vi "Find Queue (SubVI).vi"(10 "Module":string, 11 "Input":T1 {"Main Config"."PR Module Configs"."Settings"."PID 2 Parameters"."output range"."output low" format="%.2f"; "Main Config"."PR Module Configs"."Settings"."PID 2 Parameters"."output range"."output high" min=0.0 max=100.0 format="%.2f"; "Main Config"."PR Module Configs"."Settings"."PID 2 Parameters"."PID gains"."derivative time (Td, min)" format="%.3f"; "Main Config"."PR Module Configs"."Settings"."PID 2 Parameters"."PID gains"."integral time (Ti, min)" format="%.3f"; "Main Config"."PR Module Configs"."Settings"."PID 2 Parameters"."PID gains"."proportional gain (Kc)" format="%.3f"; "Main Config"."Steps"."Control" items=["Pump %", "Setpoint"]; "Main Config"."TCU Module Configs"."Settings"."Huber Unistat 410 Settings"."Address" min=0 max=99 format="%02.0f"; "Main Config"."TCU Module Configs"."Settings"."Julabo FP-50 Settings"."Pump Power" min=0 max=8 step=1; "Main Config"."TCU Module Configs"."Settings"."Lauda Settings"."Pump Power" min=0 max=8 step=1; "Main Config"."Flow Module Configs"."Settings"."Bronkhorst M14 Settings"."Smoothing Steps" min=1 step=1; "Main Config"."Flow Module Configs"."Settings"."Bronkhorst M13 Settings"."Smoothing Steps" min=1 step=1; "Main Config"."Pump Module Configs"."Settings"."Ismatech 3 Channel Settings"."Channel Number" min=0 max=3; "Main Config"."Pump Module Configs"."Settings"."Ismatech 3 Channel Settings"."Pump Number" min=1; "Main Config"."Pump Module Configs"."Settings"."ASIA Pump C"."channel" min=0 max=1 step=1; "Main Config"."Pump Module Configs"."Settings"."Masterflex"."Pump Number" min=1.0 max=20.0 step=1.0; "Main Config"."Pump Module Configs"."Settings"."Ismatech"."Pump Number" min=1.0 max=20.0 step=1.0; "Main Config"."Feed Module Configs"."Settings"."Bronkhorst M14 Settings"."Smoothing Steps" min=1 step=1; "Main Config"."Feed Module Configs"."Settings"."Ismatech 3 Channel Settings"."Channel Number" min=0 max=3; "Main Config"."Feed Module Configs"."Settings"."Ismatech 3 Channel Settings"."Pump Number" min=1; "Main Config"."Feed Module Configs"."Settings"."output range"."output low" min=0.0 max=100.0 format="%.2f"; "Main Config"."Feed Module Configs"."Settings"."output range"."output high" format="%.2f"; "Main Config"."Feed Module Configs"."Settings"."PID 2 Parameters"."PID gains"."derivative time (Td, min)" format="%.3f"; "Main Config"."Feed Module Configs"."Settings"."PID 2 Parameters"."PID gains"."integral time (Ti, min)" format="%.3f"; "Main Config"."Feed Module Configs"."Settings"."PID 2 Parameters"."PID gains"."proportional gain (Kc)" format="%.3f"; "Main Config"."Feed Module Configs"."Settings"."Bronkhorst M13 Flow Meter"."Smoothing Steps" min=1 step=1; "Main Config"."Feed Module Configs"."Settings"."ASIA Pump C"."channel" min=0 max=1 step=1; "Main Config"."Feed Module Configs"."Settings"."Ismatech"."Pump Number" min=1.0 max=20.0 step=1.0; "Main Config"."Feed Module Configs"."Settings"."Masterflex"."Pump Number" min=1.0 max=20.0 step=1.0}) -> (2 "Found?":bool, 3 "Queue out":refnum<queue>)   [LabVIEW 2018, in "Sequencing Library.lvlib"]
uses:
  Sequencing Library.lvlib
  support/Message Queue/Message Cluster.ctl
  Drag and Drop/State Cluster.ctl
  Drag and Drop/Thumbnail Cluster.ctl
  Drag and Drop/Object Cluster.ctl
  <vilib>/Utility/miscctls.llb/LVRectTypeDef.ctl
  Drag and Drop/Object Type Enum.ctl
  <vilib>/Utility/miscctls.llb/LVPositionTypeDef.ctl
  Config Module/Controls/Main Config Cluster.ctl
  OPC/OPC Module Config.ctl
  Scale Module Folder/Measure Instrument/State Enum.ctl
  <vilib>/Utility/miscctls.llb/LVPoint32TypeDef.ctl
  OPC/OPC Settings.ctl
  OPC/Variable Data Cluster.ctl
  <vilib>/OPCUA/controls/NodeId.ctl
  <vilib>/OPCUA/controls/OPC UA StatusCode.ctl
  <vilib>/OPCUA/controls/Subscription ID.ctl
  <vilib>/OPCUA/controls/OPC UA Client Refnum.ctl
  <vilib>/OPCUA/controls/Subscription Data Change.ctl
  <vilib>/OPCUA/controls/Data Type.ctl
  OPC/OPC Tag Data.ctl
  Feed Module/Controls/Feed Module Config Cluster.ctl
  Feed Module/Controls/Feed Module Settings Cluster.ctl
  Ismatec ISM 831C/Controls/Ismatech ISM831C Settings Cluster.ctl
  Masterflex 7550-30/Controls/Settings Cluster.ctl
  Mettler Toledo/Controls/Settings Cluster.ctl
  Bronkhorst M13 Flow Meter/Settings Cluster.ctl
  Measure Instrument/PID 2 Parameters Cluster.ctl
  Measure Instrument/PID Input Enum.ctl
  Measure Instrument/PID 2 Output Enum.ctl
  Tacmina QI/Tacmina QI DAQ Setting.ctl
  KNF Pump/Settings Cluster plus SIMDOS.ctl
  ASIA Pump/Pump Settings.ctl
  VICI M50 Party Mode/Settings Cluster.ctl
  FLOM Pump/Settings Cluster.ctl
  SSI PR Class/SSI PR or LD Settings Cluster.ctl
  Masterflex 75211/Masterflex 75211 DAQ Setting.ctl
  SSI PR Class/SSI P40 Settings Cluster.ctl
  Ismatec 78001/Ismatec 4083.ctl
  Bronkhorst M14 Flow Meter/Settings Cluster.ctl
  TT Module/Controls/TT Module Config Cluster.ctl
  Tag VIs/Numeric Alarm Settings Cluster.ctl
  Acquisition/Hardware Configuration.ctl
  Acquisition/Task Cluster.ctl
  PT Module/Controls/PT Module Config Cluster.ctl
  Scale Module Folder/Feed Module/Controls/Scale Module Config Cluster.ctl
  Scale Module Folder/Feed Module/Controls/Scale Module Settings Cluster.ctl
  Pump Module Folder/Pump Module Config Cluster.ctl
  Pump Module Folder/Pump Module Settings Cluster.ctl
  LabJack Module/Controls/U3 Module Config Cluster.ctl
  Decoration Module/Decoration Module Config Cluster.ctl
  Flow Module Folder/Feed Module/Controls/Flow Module Config Cluster.ctl
  Flow Module Folder/Feed Module/Controls/Flow Module Settings Cluster.ctl
  TCU Module/TCU Module Folder/TCU Module Config Cluster.ctl
  TCU Module/TCU Module Folder/TCU Module Settings Cluster.ctl
  TCU Module/TCU Module Folder/Measure Instrument/Output Devices.ctl
  Huber TCU/Huber Settings.ctl
  Lauda Integral XT-150 TCU/Lauda Settings.ctl
  Julabo Type 1 TCU/Julabo Type 1 TCU Folder/Julabo FP-50 Settings.ctl
  Huber Unistat 410 TCU/Huber Unistat 410 RS485 Settings.ctl
  D-O Module Folder/Not Sure Where this is Used.ctl
  Squence Control.ctl
  D-O Module Folder/D-O Module Config Cluster.ctl
  D-O Module Folder/Valve Clusters.ctl
  D-O Module Folder/D-O Module Settings Cluster.ctl
  D-O Module Folder/D-O Device Settings Cluster.ctl
  VICI Electronic Actuator/VICI Electronic Actuator Settings.ctl
  Pressure Regulator Control Module/Pressure Regulator/Controls/4-20mA Module Config Cluster.ctl
  Pressure Regulator Control Module/Pressure Regulator/Controls/4-20mA Module Settings Cluster.ctl
  Pressure Transmitter/Pressure Transmitter Device Settings.ctl
  Pressure Reg Module/Pressure Regulator Device Settings.ctl
  Sonicator Module Folder/Feed Module/Controls/Sonicator Module Config Cluster.ctl
  Sonicator Module Folder/Feed Module/Controls/Sonicator Module Settings Cluster.ctl
  Sonic Systems P100/Sonic Systems P100 Settings.ctl
  Agitator Module Folder - Copy/Feed Module/Controls/Agitator Module Config Cluster.ctl
  Agitator Module Folder - Copy/Feed Module/Controls/Agitator Module Settings Cluster.ctl
  support/Message Queue/Message Queue.lvlib
  TT Module/TT Module.lvlib
  Ismatec ISM 831C/Ismatec ISM 831C.lvlib
  Masterflex 7550-30/Masterflex 7550-30.lvlib
  Mettler Toledo/Mettler Toledo.lvlib
  Bronkhorst M13 Flow Meter/Bronkhorst M13 Flow Meter.lvlib
  Tacmina QI/Tacmina QI.lvlib
  KNF Pump/KNF SIMDOS.lvlib
  ASIA Pump.lvlib
  Feed Module/Feed Module.lvlib
  DAQ/DAQ.lvlib
  PT Module/PT Module.lvlib
  Scale Module Folder/Scale Module.lvlib
  Pump Module Folder/Pump Module.lvlib
  LabJack Module/U3 Module.lvlib
  Flow Module Folder/Flow Module.lvlib
  Huber TCU/Huber Ministat 230 TCU.lvlib
  Lauda Integral XT-150 TCU/Lauda TCU.lvlib
  Julabo Type 1 TCU/Julabo Type 1 TCU Folder/Julabo Type FP-50 TCU.lvlib
  TCU Module/TCU Module Folder/TCU Module.lvlib
  Config Module/Config Module.lvlib
  Drag and Drop/Drag and Drop.lvlib
  VICI M50 Party Mode/VICI M6 M50 Party Mode.lvlib
  D-O Module Folder/D-O Module.lvlib
  Pressure Transmitter/Pressure Transmitter Library.lvlib
  Pressure Regulator Control Module/Pressure Regulator/4-20mA Module.lvlib
  Pressure Reg Module/Pressure Regulator Library.lvlib
  FLOM Pump/FLOM Pump.lvlib
  SSI PR Class/SSI PR or LD Pump.lvlib
  OPC/OPC UA.lvlib
  Scale Module Folder/Measure Instrument/Scale Module Engine.lvlib
  D-O Module Folder/DIO Valve/VICI Electronic Actuator.lvlib
  Masterflex 75211/Masterflex 75211.lvlib
  SSI PR Class/SSI P40 Pump.lvlib
  Huber Unistat 410 TCU/Huber Unistat 410 TCU.lvlib
  Ismatec 78001/Ismatec 4308.lvlib
  Bronkhorst M14 Flow Meter/Bronkhorst M14 Flow Meter.lvlib
  Sonicator Module Folder/Sonicator Module.lvlib
  Sonic Systems P100/Sonic Systems P100.lvlib
  Agitator Module Folder - Copy/Agitator Module.lvlib
panel:
  # "Agitator Settings"
  # "Sonicator Settings"
  # "Instrument Settings"
  # "Instrument Settings"
  # "Output Instruments"
  # "Flow Meter Settings"
  # "Output Instruments"
  # "Scale Settings"
  # "Output Instruments"
  # "Input Instruments"
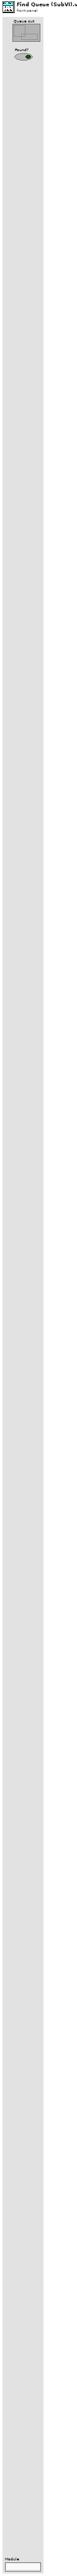
[diagram p1: front panel]
types:
  T1 = typedef "Drag and Drop.lvlib/State Cluster.ctl" = cluster{"VI refs":refnum<vi>[], "Queues":refnum<queue>[], "[Thumbnails]":T2[], "Drag Object Idx":i32, "[Objects]":T3[], "Active Object":i32, "Drop Offset":T6, "Process Name":string, "Main Config":T7, "Campaign Filepath":path, "Config Changed?":bool}
  T2 = typedef "Thumbnail Cluster.ctl" = cluster{"Path":path, "Rectangle":cluster{"left":i16, "top":i16, "right":i16, "bottom":i16}}
  T3 = typedef "Object Cluster.ctl" = cluster{"BMP Path":path, "Anchor Position":cluster{"X":i32, "Y":i32}, "Hot Spot":T4, "Type":T5, "Parameters":variant}
  T4 = typedef "LVRectTypeDef.ctl" = cluster{"Left":i16, "Top":i16, "Right":i16, "Bottom":i16}
  T5 = typedef "Object Type Enum.ctl" = enum16{"Icon", "Line", "Text", "Feed Module"}
  T6 = typedef "LVPositionTypeDef.ctl" = cluster{"Left":i32, "Top":i32}
  T7 = typedef "Config Module.lvlib/Main Config Cluster.ctl" = cluster{"Notebook":string, "OPC Module Configs":T8[], "Feed Module Configs":T18[], "Log File Path":path, "TT Module Configs":T37[], "DAQ Config":T39, "PT Module Configs":T41[], "Scale Module Configs":T42[], "Pump Module Configs":T44[], "U3 Module Configs":T46[], "Decoration Module Configs":T47[], "Flow Module Configs":T48[], "TCU Module Configs":T50[], "Steps":T57, "Abort":bool, "DO Module Configs":T59[], "PR Module Configs":T64[], "SC Module Configs":T68[], "AM Module Configs":T71[], "Cycle Period":dbl}
  T8 = typedef "OPC UA.lvlib/OPC Module Config.ctl" = cluster{"State":T9, "GUID":string, "Drop Coords":T10, "Configuration":T11, "First Iteration":bool, "Data":cluster{"Object Name":string, "Variable Array":T12[]}[], "Process Name":string, "Load Count":i32, "Log Started":bool, "subscription ID out":T15, "OPC UA client refnum out":T16, "Event Registration Refnum":refnum<event-registration>, "Start Time":timestamp, "Current Time":timestamp, "Tag Data":T17[]}
  T9 = typedef "Scale Module.lvlib/Scale Module Engine.lvlib/State Enum.ctl" = enum16{"Measuring", "Idle"}
  T10 = typedef "LVPoint32TypeDef.ctl" = cluster{"Horizontal":i32, "Vertical":i32}
  T11 = typedef "OPC UA.lvlib/OPC Settings.ctl" = cluster{"Cycle Period":dbl, "server endpoint URL":string, "security policy":cluster{"message mode":enum16{"None", "Sign", "Sign and Encrypt"}, "security":enum16{"Basic256", "Basic128Rsa15"}}, "Trust Any Server":bool}
  T12 = typedef "OPC UA.lvlib/Variable Data Cluster.ctl" = cluster{"node ID":T13, "browse name":string, "status":T14, "timestamp":timestamp, "value ":variant}
  T13 = typedef "NodeId.ctl" = string
  T14 = typedef "OPC UA StatusCode.ctl" = u32
  T15 = typedef "Subscription ID.ctl" = u32
  T16 = typedef "OPC UA Client Refnum.ctl" = refnum<k21>
  T17 = typedef "OPC UA.lvlib/OPC Tag Data.ctl" = cluster{"Include this Device":bool, "Device Name":string, "OPC Tag Data":cluster{"Tag":string, "Value":variant, "Time Stamp":timestamp}[]}
  T18 = typedef "Feed Module.lvlib/Feed Module Config Cluster.ctl" = cluster{"GUID":string, "Drop Coords":T10, "Process Name":string, "Queue Name":string, "Settings":T19, "Settings Load Count":i32, "OP Load Count":i32}
  T19 = typedef "Feed Module.lvlib/Feed Module Settings Cluster.ctl" = cluster{"Cycle Period":dbl, "Ismatech":T20, "Masterflex":T21, "Mettler":T22, "Bronkhorst M13 Flow Meter":T23, "PID 2 Parameters":T24, "Manual Entry":dbl, "Auto?":bool, "output range":cluster{"output high":dbl, "output low":dbl}, "Tacmina Settings":T27, "KNF SIMDOS Settings":T28, "ASIA Pump C":T29, "VICI Settings":T30, "FLOM Settings":T31, "SSI PR/LD Settings":T32, "Masterflex 75211 Settings":T33, "SSI P40 Settings":T34, "Ismatech 3 Channel Settings":T35, "Bronkhorst M14 Settings":T36}
  T20 = typedef "Ismatec ISM 831C.lvlib/Ismatech ISM831C Settings Cluster.ctl" = cluster{"VISA resource name":refnum<visa-resource-name>, "Simulated?":bool, "Pump Number":dbl, "Reverse?":bool}
  T21 = typedef "Masterflex 7550-30.lvlib/Settings Cluster.ctl" = cluster{"VISA resource name":refnum<visa-resource-name>, "Simulated?":bool, "Pump Number":dbl, "Reverse?":bool}
  T22 = typedef "Mettler Toledo.lvlib/Settings Cluster.ctl" = cluster{"VISA resource name":refnum<visa-resource-name>, "Simulated?":bool}
  T23 = typedef "Bronkhorst M13 Flow Meter.lvlib/Settings Cluster.ctl" = cluster{"VISA resource name":refnum<visa-resource-name>, "Simulated?":bool, "Smoothing Steps":i32}
  T24 = typedef "PID 2 Parameters Cluster.ctl" = cluster{"Input Device":T25, "Output Device":T26, "Setpoint":dbl, "PID gains":cluster{"proportional gain (Kc)":dbl, "integral time (Ti, min)":dbl, "derivative time (Td, min)":dbl}}
  T25 = typedef "PID Input Enum.ctl" = enum16{"Default", "Bronkhorst M13", "Bronkhorst M14", "Scale Rate of Change"}
  T26 = typedef "PID 2 Output Enum.ctl" = enum16{"Default", "Ismatec ISM 4308", "Ismatec ISM 831C", "Masterflex 7550-30", "VICI", "Tacmina QI", "KNF SIMDOS", "ASIA Type C", "FLOM UI-22-11", "SSI PR/LD", "SSI P40", "Masterflex 75211-70"}
  T27 = typedef "Tacmina QI.lvlib/Tacmina QI DAQ Setting.ctl" = cluster{"Analog DAQ Task":refnum<k21>, "Digital DAQ Task":refnum<k21>}
  T28 = typedef "KNF SIMDOS.lvlib/Settings Cluster plus SIMDOS.ctl" = cluster{"VISA resource name":refnum<visa-resource-name>, "Simulated?":bool}
  T29 = typedef "ASIA Pump.lvlib/Pump Settings.ctl" = cluster{"ASIA Pump #":i32, "channel":i32, "Simulated":bool}
  T30 = typedef "VICI M6 M50 Party Mode.lvlib/Settings Cluster.ctl" = cluster{"VISA resource name":refnum<visa-resource-name>, "Simulated?":bool, "Pump Letter":string, "Reverse?":bool}
  T31 = typedef "FLOM Pump.lvlib/Settings Cluster.ctl" = cluster{"VISA resource name":refnum<visa-resource-name>, "Simulated?":bool, "Pump Number":dbl}
  T32 = typedef "SSI PR or LD Pump.lvlib/SSI PR or LD Settings Cluster.ctl" = cluster{"VISA resource name":refnum<visa-resource-name>, "Simulated?":bool}
  T33 = typedef "Masterflex 75211.lvlib/Masterflex 75211 DAQ Setting.ctl" = cluster{"Analog DAQ Task":refnum<k21>, "Digital DAQ Task":refnum<k21>}
  T34 = typedef "SSI P40 Pump.lvlib/SSI P40 Settings Cluster.ctl" = cluster{"VISA resource name":refnum<visa-resource-name>, "Simulated?":bool}
  T35 = typedef "Ismatec 4308.lvlib/Ismatec 4083.ctl" = cluster{"VISA resource name":refnum<visa-resource-name>, "Pump Number":i16, "Channel Number":i16, "Simulated?":bool, "Reverse?":bool}
  T36 = typedef "Bronkhorst M14 Flow Meter.lvlib/Settings Cluster.ctl" = cluster{"VISA resource name":refnum<visa-resource-name>, "Simulated?":bool, "Smoothing Steps":i32}
  T37 = typedef "TT Module.lvlib/TT Module Config Cluster.ctl" = cluster{"GUID":string, "Drop Coords":T10, "Input Channel Tag Name ":string, "Process Name":string, "Queue Name":string, "Input Channel Numeric Alarm Settings":T38[]}
  T38 = typedef "Numeric Alarm Settings Cluster.ctl" = cluster{"enable? (F)":bool, "name":string, "alarm type":enum16{"HI_HI", "HI", "LO", "LO_LO"}, "level/change":dbl, "deadband/time":dbl, "alarm delay":dbl, "priority":u32, "ack type":enum16{"Auto", "User", "None", "Each Occurrence"}, "area":string, "description":string, "log? (T)":bool}
  T39 = typedef "DAQ.lvlib/Hardware Configuration.ctl" = cluster{"Tasks":T40[]}
  T40 = typedef "Task Cluster.ctl" = cluster{"DAQmx Task":refnum<k21>, "Read-Write Radio":enum32{"Read", "Write"}}
  T41 = typedef "PT Module.lvlib/PT Module Config Cluster.ctl" = cluster{"GUID":string, "Drop Coords":T10, "Input Channel Tag Name ":string, "Process Name":string, "Queue Name":string, "Input Channel Numeric Alarm Settings":T38[]}
  T42 = typedef "Scale Module.lvlib/Scale Module Config Cluster.ctl" = cluster{"GUID":string, "Drop Coords":T10, "Process Name":string, "Queue Name":string, "Settings":T43, "Load Count":i32}
  T43 = typedef "Scale Module.lvlib/Scale Module Settings Cluster.ctl" = cluster{"Cycle Period":dbl, "Mettler":T22, "Scale Type":string}
  T44 = typedef "Pump Module.lvlib/Pump Module Config Cluster.ctl" = cluster{"GUID":string, "Drop Coords":T10, "Process Name":string, "Queue Name":string, "Settings":T45, "Load Count":i32}
  T45 = typedef "Pump Module.lvlib/Pump Module Settings Cluster.ctl" = cluster{"Cycle Period":dbl, "Manual Entry":dbl, "Output Device":T26, "Ismatech":T20, "Ismatech 3 Channel Settings":T35, "Masterflex":T21, "VICI Settings":T30, "Tacmina Settings":T27, "KNF SIMDOS Settings":T28, "ASIA Pump C":T29, "FLOM Settings":T31, "SSI PR/LD Settings":T32, "SSI P40 Settings":T32, "Masterflex 75211 Settings":T33, "Pump Calibration File":path, "Calibration Slope":dbl, "Calibration Y Intercept":dbl, "Pump Cal Enum":u16}
  T46 = typedef "U3 Module.lvlib/U3 Module Config Cluster.ctl" = cluster{"GUID":string, "Drop Coords":T10, "AI Channel Number":enum16{"Default", "AI0", "AI1", "AI2", "AI3", "AI4", "AI5", "AI6", "AI7"}, "Process Name":string, "Queue Name":string, "Input Channel Numeric Alarm Settings":T38[]}
  T47 = typedef "Decoration Module Config Cluster.ctl" = cluster{"GUID":string, "Drop Coords":T10, "Decoration Filepath":path}
  T48 = typedef "Flow Module.lvlib/Flow Module Config Cluster.ctl" = cluster{"GUID":string, "Drop Coords":T10, "Process Name":string, "Queue Name":string, "Settings":T49, "Load Count":i32}
  T49 = typedef "Flow Module.lvlib/Flow Module Settings Cluster.ctl" = cluster{"Cycle Period":dbl, "Flow Meter Type":string, "Bronkhorst M13 Settings":T23, "Bronkhorst M14 Settings":T36}
  T50 = typedef "TCU Module.lvlib/TCU Module Config Cluster.ctl" = cluster{"GUID":string, "Drop Coords":T10, "Process Name":string, "Queue Name":string, "Settings":T51, "Load Count":i32, "Power Level Changed":bool}
  T51 = typedef "TCU Module.lvlib/TCU Module Settings Cluster.ctl" = cluster{"Cycle Period":dbl, "Setpoint Entry":dbl, "Output Device":T52, "Huber Ministat 230 Settings":T53, "Lauda Settings":T54, "Julabo FP-50 Settings":T55, "Internal Control?":bool, "Huber Unistat 410 Settings":T56}
  T52 = typedef "Output Devices.ctl" = enum16{"Default", "Huber Ministat 230", "Huber Unistat 410", "Lauda XT-150", "Julabo FP-50"}
  T53 = typedef "Huber Ministat 230 TCU.lvlib/Huber Settings.ctl" = cluster{"VISA resource name":refnum<visa-resource-name>, "Simulated?":bool}
  T54 = typedef "Lauda TCU.lvlib/Lauda Settings.ctl" = cluster{"VISA resource name":refnum<visa-resource-name>, "Simulated?":bool, "Pump Power":i32}
  T55 = typedef "Julabo Type FP-50 TCU.lvlib/Julabo FP-50 Settings.ctl" = cluster{"VISA resource name":refnum<visa-resource-name>, "Simulated?":bool, "Pump Power":i32}
  T56 = typedef "Huber Unistat 410 TCU.lvlib/Huber Unistat 410 RS485 Settings.ctl" = cluster{"VISA resource name":refnum<visa-resource-name>, "Address":i8, "Simulated?":bool}
  T57 = typedef "Not Sure Where this is Used.ctl" = T58[]
  T58 = typedef "Sequencing Library.lvlib/Squence Control.ctl" = cluster{"Module":string, "Control":u16, "Value":dbl, "Wait (sec)":dbl}
  T59 = typedef "D-O Module.lvlib/D-O Module Config Cluster.ctl" = cluster{"GUID":string, "Drop Coords":T10, "Process Name":string, "Queue Name":string, "Settings":T60, "Load Count":i32}
  T60 = typedef "D-O Module.lvlib/Valve Clusters.ctl" = cluster{"Valve Settings":T61, "Valve Type":enum16{"Default", "Digital Output Valve", "VICI Electronic Actuator"}, "Time On (Sec)":dbl, "Time Off (Sec)":dbl, "Run?":bool}
  T61 = typedef "D-O Module.lvlib/D-O Module Settings Cluster.ctl" = cluster{"D-O Settings":T62, "VICI Electronic Actuator":T63}
  T62 = typedef "D-O Module.lvlib/D-O Device Settings Cluster.ctl" = cluster{"DAQmx Task Name":refnum<k21>, "Output Channel":u16, "Output Channel Names":string[]}
  T63 = typedef "VICI Electronic Actuator.lvlib/VICI Electronic Actuator Settings.ctl" = cluster{"VISA resource name":refnum<visa-resource-name>, "Mode":enum16{"Two Positions With Stops", "Two Positions Without Stops", "Mutiposition"}, "Simulated":bool}
  T64 = typedef "4-20mA Module.lvlib/4-20mA Module Config Cluster.ctl" = cluster{"GUID":string, "Drop Coords":T10, "Process Name":string, "Queue Name":string, "Settings":T65, "Settings Load Count":i32}
  T65 = typedef "4-20mA Module.lvlib/4-20mA Module Settings Cluster.ctl" = cluster{"Cycle Period":dbl, "PID 2 Parameters":cluster{"Input Device":enum16{"Default", "4-20mA"}, "Output Device":enum16{"Default", "Equilibar Pressure Reg", "Flow Regulator"}, "Setpoint":dbl, "PID gains":cluster{"proportional gain (Kc)":dbl, "integral time (Ti, min)":dbl, "derivative time (Td, min)":dbl}, "output range":cluster{"output low":dbl, "output high":dbl}}, "Manual Entry":dbl, "Auto?":bool, "4-20mA Input Settings":T66, "4-20mA Out Settings":T67, "Input Channel Tag Name ":string}
  T66 = typedef "Pressure Transmitter Library.lvlib/Pressure Transmitter Device Settings.ctl" = cluster{"Input Channel ":u16}
  T67 = typedef "Pressure Regulator Library.lvlib/Pressure Regulator Device Settings.ctl" = cluster{"Output DAQ Task":refnum<k21>}
  T68 = typedef "Sonicator Module.lvlib/Sonicator Module Config Cluster.ctl" = cluster{"GUID":string, "Drop Coords":T10, "Process Name":string, "Queue Name":string, "Settings":T69, "Load Count":i32}
  T69 = typedef "Sonicator Module.lvlib/Sonicator Module Settings Cluster.ctl" = cluster{"Cycle Period":dbl, "Sonicator Type":string, "SS P100 Settings":T70, "Setpoint (µm)":dbl, "Cutoff (µm)":dbl}
  T70 = typedef "Sonic Systems P100.lvlib/Sonic Systems P100 Settings.ctl" = cluster{"VISA resource name":refnum<visa-resource-name>, "Simulated?":bool}
  T71 = typedef "Agitator Module.lvlib/Agitator Module Config Cluster.ctl" = cluster{"GUID":string, "Drop Coords":T10, "Process Name":string, "Queue Name":string, "Settings":T72, "Load Count":i32}
  T72 = typedef "Agitator Module.lvlib/Agitator Module Settings Cluster.ctl" = cluster{"Cycle Period":dbl, "Agitator Type":string, "Setpoint (µm)":dbl}
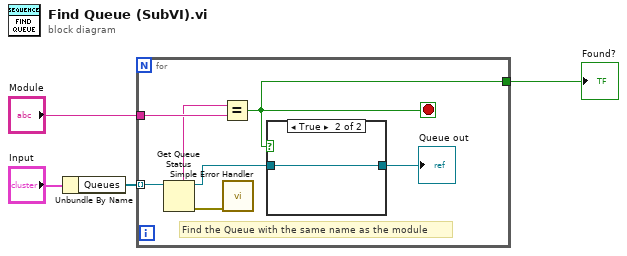
[diagram p0: block diagram]
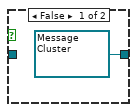
[diagram p2: hidden frame]
diagram:
  n1 = Unbundle By Name("Input") -> ("Queues"=w4:refnum<queue>[])
  n2 = for {
    tunnel: "Module" -> [w11]
    tunnel: [w5] -> w2
    tunnel: w4 -> [w9] mode=indexing
    stop <- w5 stop-if-true
    # "Find the Queue with the same name as the module"
    n3 = Get Queue Status(queue=w9) -> (queue out=w8:refnum<queue>, queue name=w10:string, error out=w6:errorcluster)  [unwired: 2 in, 5 out]
    n4 = Equal?(x=w10, y=w11) -> (x = y?=w5:bool)
    n5 = call <vilib>:"Simple Error Handler.vi"("error in (no error)"=w6) -> ()  [unwired: 4 in, 5 out]
    n6 = case shown="True" w5 {
      tunnel: w8 -> [_ w13]
      tunnel: [refnum<queue> refnum ("Message Queue") w13] -> w7
      frame False {
      }
      frame True {
      }
    }
    "Queue out" <- w7
  }
  "Found?" <- w2
